vi "edittest parse query params.vi"(11 "ENV":T1) -> (0 "Client Address":string, 1 "First Value":string, 2 "First Key":string, 3 "Query Parameters":T1)   [LabVIEW 2011]
uses:
  ITK EXT/utils/keyedarr.llb/Keyed Array.ctl
  ITK EXT/utils/strutil.llb/Case Matching.ctl
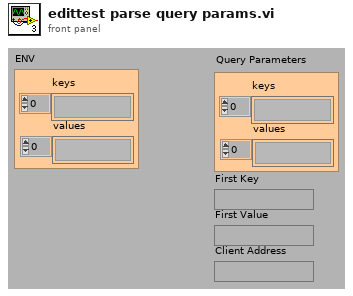
[diagram p1: front panel]
types:
  T1 = typedef "Keyed Array.ctl" = cluster{"keys":string[], "values":string[]}
  T2 = typedef "Case Matching.ctl" = enum16{"a != A", "a == A", "system"}
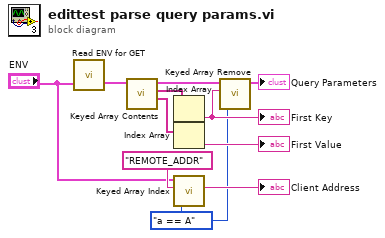
[diagram p0: block diagram]
diagram:
  w3 = Case_Matching."a == A" ("case matching (sensitive)")
  n1 = call "Read ENV for GET.vi"("ENV"="ENV") -> ("GET query params"=w2:T1)  [unwired: 2 out]
  n2 = call "Keyed Array Contents.vi"("array in"=w2) -> ("values"=w8:string[], "keys"=w11:string[], "duplicate array"=w10:T1)  [unwired: 4 out]
  n3 = Index Array(array=w11) -> (element=w7:string)  [unwired: 1 in]
  "First Key" <- w7
  n4 = Index Array(array=w8) -> (element=→"First Value":string)  [unwired: 1 in]
  n5 = call "Keyed Array Index.vi"("case matching (sensitive)"=w3, "key"="REMOTE_ADDR", "array in"="ENV") -> ("value"=→"Client Address":string)  [unwired: 1 in, 3 out]
  n6 = call "Keyed Array Remove.vi"("case matching (sensitive)"=w3, "key"=w7, "array in"=w10) -> ("array out"=→"Query Parameters":T1)  [unwired: 4 out]
